vi "1 Tap 16-Bit.vi"() -> (0 "PixelData":u16)   [LabVIEW 2014]
uses:
  <vilib>/rvi/eio/common/nirviEmuTemplateMethod_errors.vi
  <vilib>/eio/EIONode/EIONode.xnode
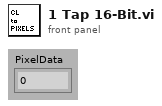
[diagram p1: front panel]
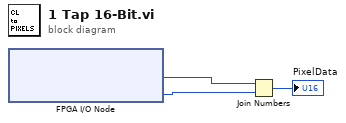
[diagram p0: block diagram]
diagram:
  n1 = xnode "FPGA I/O Node"() -> ("IO Module\\CL Port B"=w1:u8, "IO Module\\CL Port A"=w3:u8)  [unwired: 2 in, 2 out]
  n2 = Join Numbers(hi=w1, lo=w3) -> ((hi.lo)=→"PixelData":u16)
